vi "Setup - create temp root.vi"(8 "error in (no error)":errorcluster) -> (0 "error out":errorcluster, 3 "tempRoot":path)   [LabVIEW 2026, in "Tests.lvlib"]
doc: "Creates a unique temporary root folder (system temp + a Lumberjack-test-unique name) so file appenders never touch shared locations and runs are repeatable. Generalizes Logger's \"Before File Logging.\" Returns the folder path for the test and its TearDown."
uses:
  Tests.lvlib
  <vilib>/Utility/sysdir.llb/System Directory Type.ctl
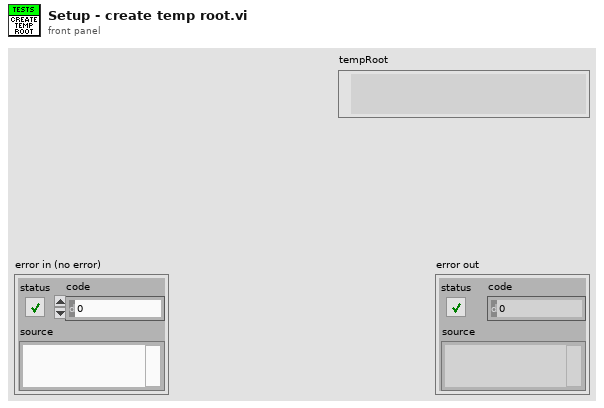
[diagram p1: front panel]
types:
  T1 = typedef "System Directory Type.ctl" = i32
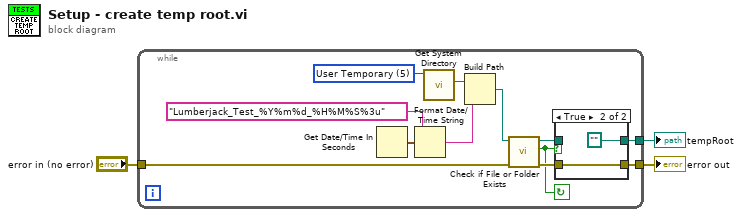
[diagram p0: block diagram]
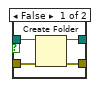
[diagram p2: hidden frame]
diagram:
  n1 = while {
    tunnel: [w5] -> w2
    tunnel: "error in (no error)" -> [w9]
    tunnel: [w13] -> w3
    stop <- w4 continue-if-true
    w15 = T1 5 items=["User Home"=0, "User Desktop"=1, "User Documents"=2, "User Application Data"=3, "User Preferences"=4, "User Temporary"=5, "Public Documents"=6, "Public Application Data"=7, "Public Preferences"=8, "Public Cache"=13, "System Core Libraries"=9, "System Installed Libraries"=10, "Application Files"=11, "Boot Volume Root"=12] ("system directory type")
    n2 = Get Date/Time In Seconds() -> (seconds since 1Jan1904=w12:timestamp)
    n3 = Format Date/Time String(time format string (%c)="Lumberjack_Test_%Y%m%d_%H%M%S%3u", seconds (now)=w12) -> (date/time string=w10:string)  [unwired: 1 in]
    n4 = call <vilib>:"Get System Directory.vi"("system directory type"=w15) -> ("system directory"=w14:path)  [unwired: 10 in]
    n5 = Build Path(base path=w14, name or relative path=w10) -> (appended path=w7:path)
    n6 = call <vilib>:"Check if File or Folder Exists.vi"("error in (no error)"=w9, "path"=w7) -> ("error out"=w8:errorcluster, "file or folder exists?"=w4:bool, "dup path"=w6:path)  [unwired: 7 in]
    n7 = case shown="True" w4 {
      tunnel: [w19 w21] -> w13
      tunnel: w6 -> [w18 _]
      tunnel: w8 -> [w17 w21]
      tunnel: [w16 path ""] -> w5
      frame False {
        n8 = Create Folder(path (use dialog)=w18, error in=w17) -> (created path=w16:path, error out=w19:errorcluster)  [unwired: 1 in, 1 out]
      }
      frame True {
      }
    }
  }
  "error out" <- w3
  "tempRoot" <- w2
